vi "Convert XLS Coordinate.vi"(11 "Excel coordinate":string) -> (1 "Column":i32, 3 "Row":i32)   [LabVIEW 2021, in "Files.lvlib"]
uses:
  Files.lvlib
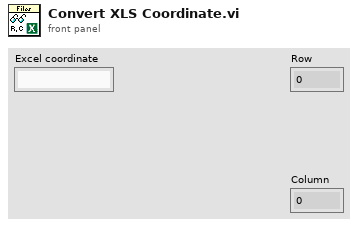
[diagram p1: front panel]
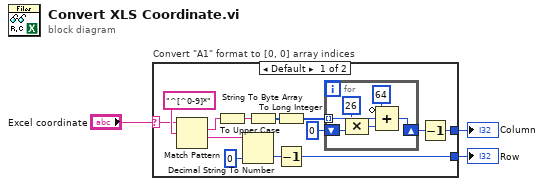
[diagram p0: block diagram]
diagram:
  n1 = case "Convert \"A1\" format to [0, 0] array indices" shown="Default" "Excel coordinate" {
    selector: "Excel coordinate" -> [w11 _]
    tunnel: [w7 _] -> w3
    tunnel: [w9 _] -> w2
    frame Default {
      n2 = Match Pattern(string=w11, regular expression="^[^0-9]*") -> (match substring=w13:string, after substring=w6:string)  [unwired: 1 in, 2 out]
      n3 = To Upper Case(1:w13) -> (0:w8:string)
      n4 = Decimal String To Number(string=w6, default (0L)=0) -> (number=w4:i32)  [unwired: 1 in, 1 out]
      n5 = String To Byte Array(string=w8) -> (unsigned byte array=w15:u8[])
      n6 = To Long Integer(number=w15) -> (32bit integer=w12:i32[])
      n7 = Decrement(x=w4) -> (x-1=w9:i32)
      n8 = for {
        tunnel: w12 -> [w22] mode=indexing
        shift-right: [w19] -> w14
        shift-left: 0 -> [w18]
        n9 = Compound Arithmetic op=MULTIPLY(26, w18) -> (w17:i32)
        n10 = Compound Arithmetic op=ADD(invert 64, w22, w17) -> (w19:i32)
      }
      n11 = Decrement(x=w14) -> (x-1=w7:i32)
    }
    frame "" {
    }
  }
  "Column" <- w3
  "Row" <- w2
